vi "ProjectionExp_H.vi"() -> ()   [LabVIEW 2017]
uses:
  <vilib>/gmath/statdist.llb/Random Permutation.vi
  <instrlib>/Tektronix TDS 200 1000 2000 Series/Tektronix TDS 200 1000 2000 Series.lvlib
  <vilib>/gmath/NI_Gmath.lvlib
panel:
  out "RandRows":i32[](array[numeric])
  out "Bernoulli random numbers":u32[](array[numeric])
  out "error 2":i32
  in  "reset":bool
  in  "seed":i32=-1
  out "Phi zeros":dbl[][](array[numeric])
  out "x2 zeros":dbl[][](array[numeric])
  out "x1 zeros":dbl[][](array[numeric])
  in  "n":i32
  out "Theta zeros":dbl[][](array[numeric])
  in  "m":i32
  out "y zeros":dbl[][](array[numeric])
  out "error out 3":errorcluster caption="error out"
  in  "Delay Time (s) 2":dbl=1.0 caption="Delay Time (s)"
  in  "error in (no error) 3":errorcluster caption="error in (no error)"
  out "error out 2":errorcluster caption="error out"
  in  "Delay Time (s)":dbl=1.0
  in  "error in (no error) 2":errorcluster caption="error in (no error)"
  out "Iteration":i32
  out "Phi":dbl[][](array[numeric])
  out "y (Measurement \nMatrix)":dbl[][](array[numeric])
  out "VISA resource name out":refnum<visa-resource-name>
  out "Measurement":dbl
  out "Units":string
  out "error out":errorcluster
  in  "VISA resource name":refnum<visa-resource-name>
  in  "Channel (1: Channel 1)":i32(ring)=1 items=["Channel 1"=1, "Channel 2"=2, "Channel 3"=3, "Channel 4"=4]
  in  "Measurement Type (0: Frequency)":i32(ring) items=["Frequency", "Mean", "Period", "Pulse Duty", "Peak to Peak", "Cycle RMS", "Minimum", "Maximum", "Rise Time", "Fall Time", "Positive Width", "Negative Width", "Amplitude", "Cycle Mean", "High", "Low", "Negative Duty", "Positive Overshoot", "Negative Overshoot", "Cursor Mean", "Burst Width", "Positive Pulse Count", "Negative Pulse Count", "Rising Edge Count", "Falling Edge Count", "Area", "Cycle Area", "RMS", "Cursor RMS"]
  in  "error in (no error)":errorcluster
  out "Theta":dbl[][](array[numeric])
  in  "k":dbl
  in  "m":dbl
  in  "n":dbl
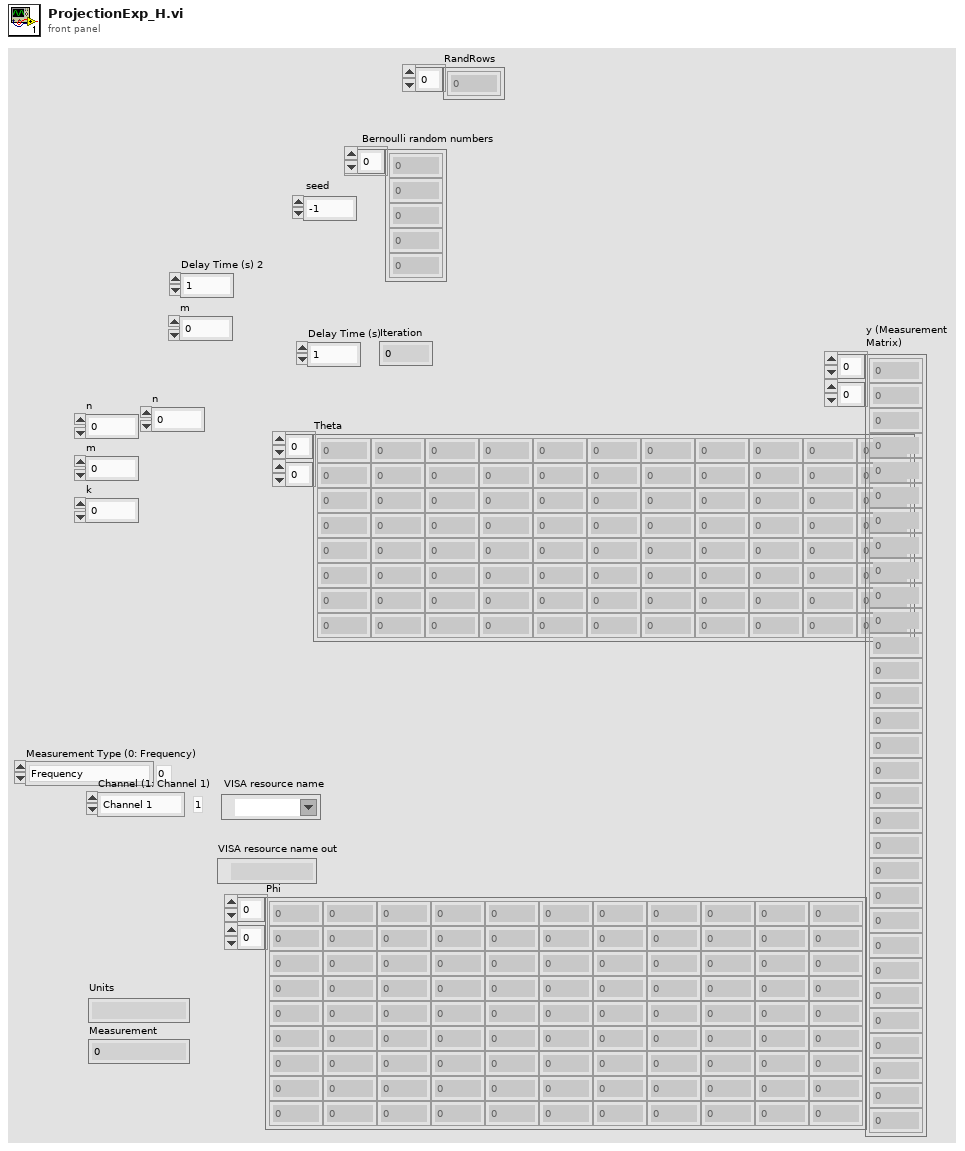
[diagram p1: front panel]
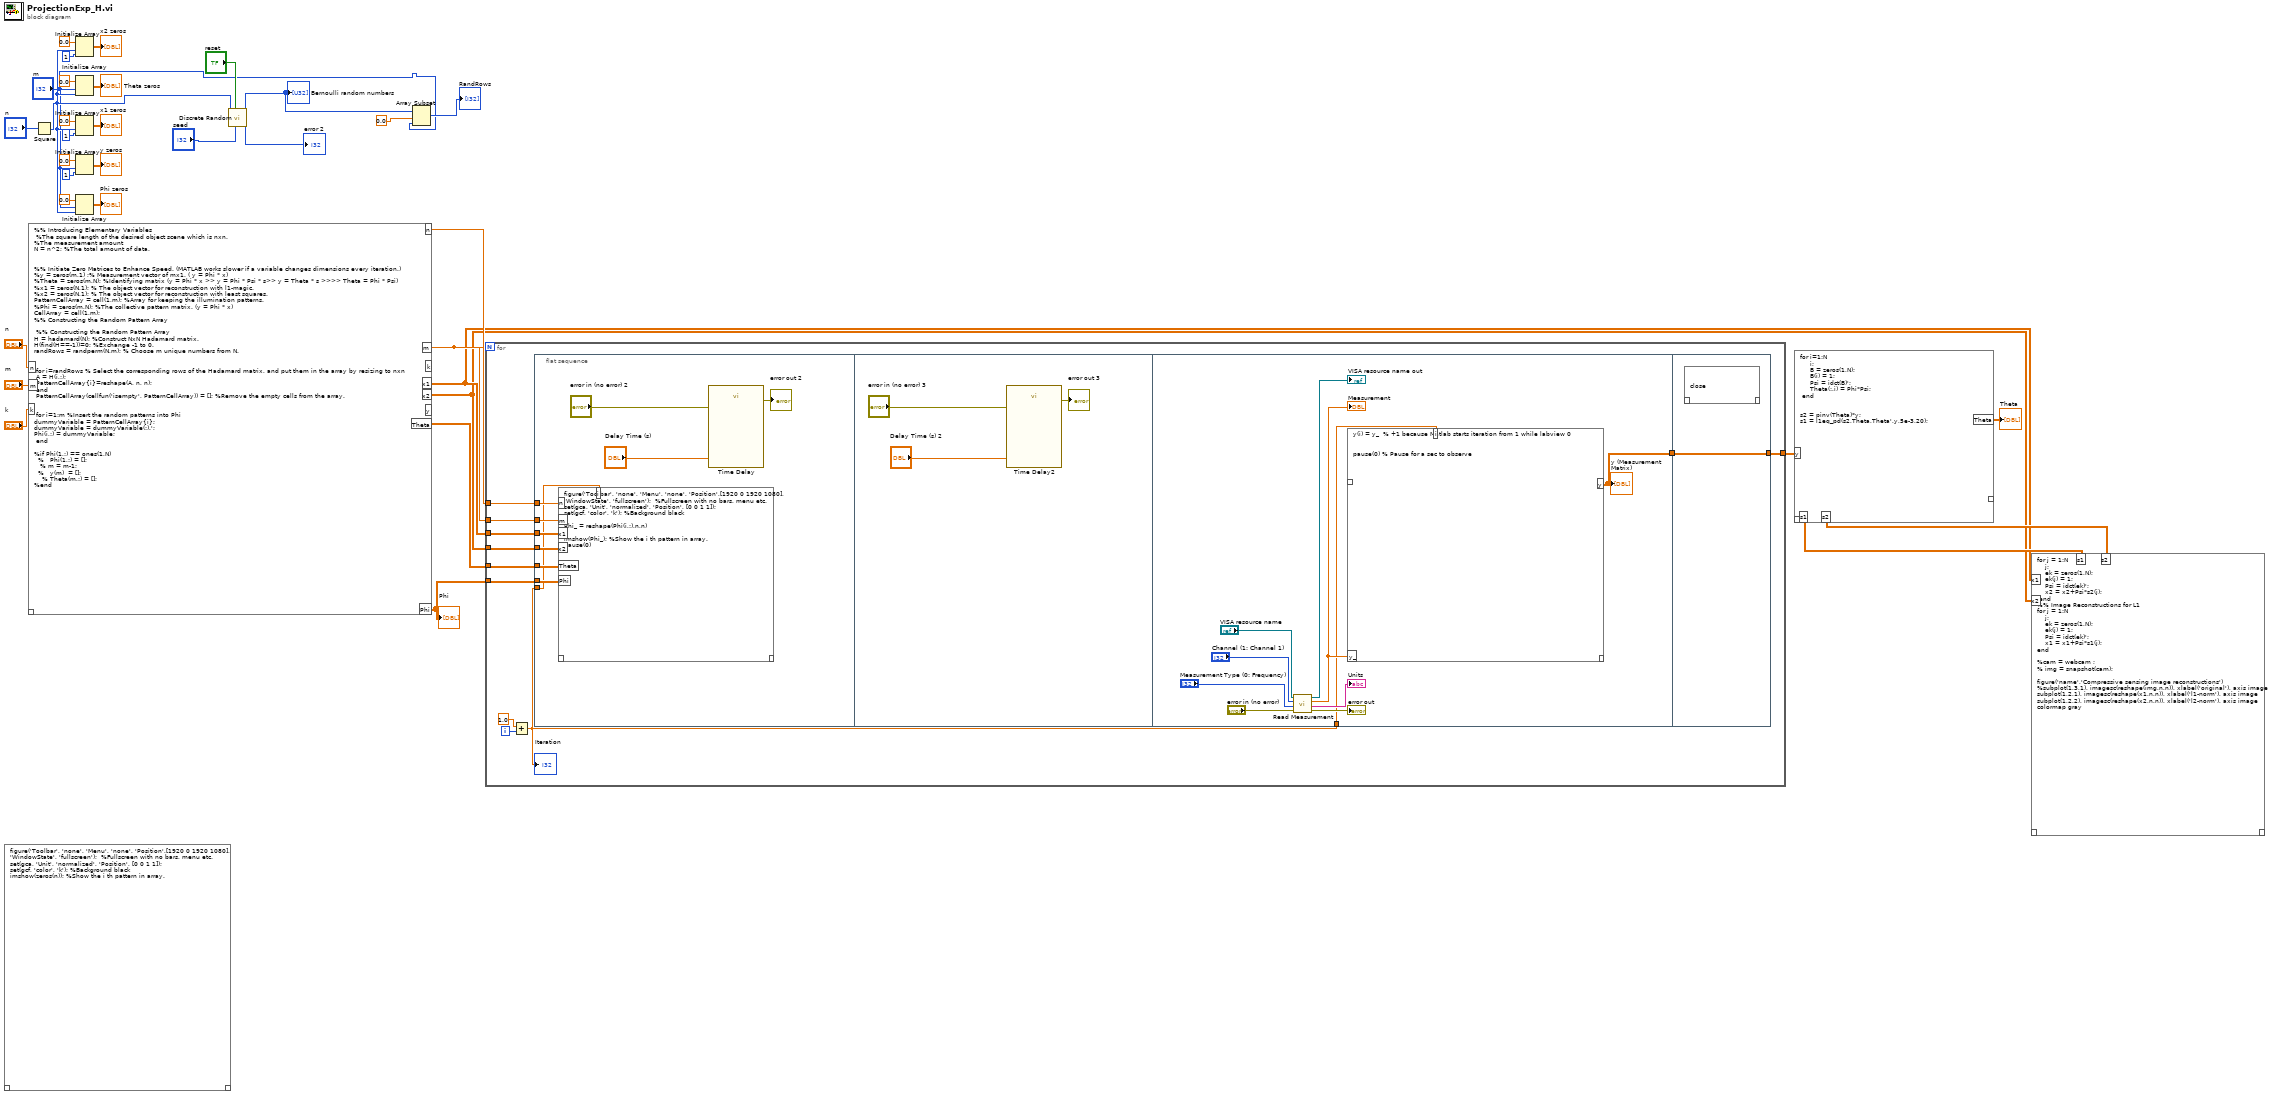
[diagram p0: block diagram]
diagram:
  n1 = script code="figure('Toolbar', 'none', 'Menu', 'none', 'Position',[1920 0 1920 1080], 'WindowState', 'fullscreen');  %Fullscreen with no bars, menu etc.\nset(gca, 'Unit', 'normalized', 'Position', [0 0 1 1]);\nset(gcf, 'color', 'k'); %Background black\nimshow(zeros(n)); %Show the i th pattern in array."() -> ()  [unwired: 1 in, 1 out]
  n2 = script code="%% Introducing Elementary Variables\n %The square length of the desired object scene which is nxn. \n%The measurement amount\nN = n^2; %The total amount of data. \n\n\n%% Initiate Zero Matrices to Enhance Speed. (MATLAB works slower if a variable changes dimensions every iteration.)\n%y = zeros(m,1) ;% Measurement vector of mx1. ( y = Phi * x)\n%Theta = zeros(m,N); %Identifying matrix (y = Phi * x >> y = Phi * Psi * s>> y = Theta * s >>>> Theta = Phi * Psi)\n%x1 = zeros(N,1); % The object vector for reconstruction with l1-magic.\n%x2 = zeros(N,1); % The object vector for reconstruction with least squares.\nPatternCellArray = cell(1,m); %Array for keeping the illumination patterns.\n%Phi = zeros(m,N); %The collective pattern matrix. (y = Phi * x)\nCellArray = cell(1,m);\n%% Constructing the Random Pattern Array\n\n %% Constructing the Random Pattern Array\nH = hadamard(N); %Construct NxN Hadamard matrix. \nH(find(H==-1))=0; %Exchange -1 to 0.\nrandRows = randperm(N,m); % Choose m unique numbers from N.\n\n\n for i=randRows % Select the corresponding rows of the Hadamard matrix, and put them in the array by resizing to nxn\n A = H(i,:);\n PatternCellArray{i}=reshape(A, n, n);\n end\n PatternCellArray(cellfun('isempty', PatternCellArray)) = []; %Remove the empty cells from the array.\n\n\n for i=1:m %Insert the random patterns into Phi\ndummyVariable = PatternCellArray{i}; \ndummyVariable = dummyVariable(:).';\nPhi(i,:) = dummyVariable;\n end\n\n%if Phi(1,:) == ones(1,N)\n  %   Phi(1,:) = [];\n   % m = m-1;\n  %   y(m)  = []; \n    % Theta(m,:) = [];\n%end"("n"="n", "m"="m", "k"="k") -> ("n"=w28:dbl, "m"=w27:dbl, "Phi"=w23:dbl[][], "Theta"=w24:dbl[][], "x1"=w26:dbl[][], "x2"=w25:dbl[][])  [unwired: 1 in, 3 out]
  "Phi" <- w23
  n3 = Square(x="n") -> (x^2=w5:i32)
  n4 = Initialize Array(0.0 ("element"), w5, 1 ("dimension size")) -> (→"x2 zeros":dbl[][])
  n5 = Initialize Array(0.0 ("element"), "m", w5) -> (→"Theta zeros":dbl[][])
  n6 = Initialize Array(0.0 ("element"), w5, 1 ("dimension size")) -> (→"x1 zeros":dbl[][])
  n7 = Initialize Array(0.0 ("element"), "m", 1 ("dimension size")) -> (→"y zeros":dbl[][])
  n8 = Initialize Array(0.0 ("element"), "m", w5) -> (→"Phi zeros":dbl[][])
  n9 = call-poly <vilib>:"Discrete Random.vi"("seed"="seed", "reset"="reset", "N"=w5) -> ("error"=→"error 2":i32, "random permutation"=w4:i32[])  [unwired: 7 in]
  "Bernoulli random numbers" <- w4
  n10 = Array Subset(array=w4, index=0.0 ("element"), length="m") -> (→"RandRows":i32[])
  n11 = for {
    N: w27 -> [_]
    tunnel: [w46] -> w29
    tunnel: w28 -> [w45]
    tunnel: w27 -> [w44]
    tunnel: w26 -> [w43]
    tunnel: w25 -> [w42]
    tunnel: w24 -> [w41]
    tunnel: w23 -> [w40]
    i -> [w37]
    n12 = Add(x=1.0, y=w37) -> (x+y=w36:dbl)
    "Iteration" <- w36
    n13 = flat-sequence {
      tunnel: w45 -> [w56]
      tunnel: w44 -> [w55]
      tunnel: w43 -> [w54]
      tunnel: w42 -> [w53]
      tunnel: w41 -> [w52]
      tunnel: w40 -> [w51]
      tunnel: w36 -> [w50]
      tunnel: w36 -> [w60]
      tunnel: [w61] -> w39
      tunnel: [w70] -> w46
      tunnel: w39 -> [w70]
      frame #0 {
        n14 = script code="figure('Toolbar', 'none', 'Menu', 'none', 'Position',[1920 0 1920 1080], 'WindowState', 'fullscreen');  %Fullscreen with no bars, menu etc.\nset(gca, 'Unit', 'normalized', 'Position', [0 0 1 1]);\nset(gcf, 'color', 'k'); %Background black\n\nPhi_ = reshape(Phi(i,:),n,n)\n\nimshow(Phi_); %Show the i th pattern in array. \npause(0)"("n"=w56, "m"=w55, "x1"=w54, "x2"=w53, "Theta"=w52, "Phi"=w51, "i"=w50) -> ()  [unwired: 1 in, 1 out]
        n15 = call "Time Delay"("error in (no error)"="error in (no error) 2", "Delay Time (s)"="Delay Time (s)") -> ("error out"=→"error out 2":errorcluster)  [unwired: 9 in]
      }
      frame #1 {
        n16 = call "Time Delay2"("error in (no error)"="error in (no error) 3", "Delay Time (s)"="Delay Time (s) 2") -> ("error out"=→"error out 3":errorcluster)  [unwired: 9 in]
      }
      frame #2 {
        n17 = call <instrlib>:"Read Measurement.vi"("error in (no error)"="error in (no error)", "Measurement Type (0: Frequency)"="Measurement Type (0: Frequency)", "Channel (1: Channel 1)"="Channel (1: Channel 1)", "VISA resource name"="VISA resource name") -> ("error out"=→"error out":errorcluster, "Units"=→"Units":string, "Measurement"=w69:dbl, "VISA resource name out"=→"VISA resource name out":refnum<visa-resource-name>)  [unwired: 4 in]
        "Measurement" <- w69
        n18 = script code="y(i) = y_  % +1 because Matlab starts iteration from 1 while labview 0 \n\n\npause(0) % Pause for a sec to observe"("i"=w60, "y_"=w69) -> ("y"=w61:dbl[][])  [unwired: 1 in, 1 out]
        "y (Measurement \nMatrix)" <- w61
      }
      frame #3 {
        n19 = script code="close"() -> ()  [unwired: 1 in, 1 out]
      }
    }
  }
  n20 = script code="for i=1:N\n     i;\n     B = zeros(1,N);\n     B(i) = 1;\n     Psi = idct(B)';\n     Theta(:,i) = Phi*Psi;    \n end\n\n\ns2 = pinv(Theta)*y;\ns1 = l1eq_pd(s2,Theta,Theta',y,5e-3,20);"("y"=w29) -> ("Theta"=→"Theta":dbl[][], "s1"=w31:dbl[][], "s2"=w30:dbl[][])  [unwired: 1 in, 1 out]
  n21 = script code="for j = 1:N\n    j;\n    ek = zeros(1,N);\n    ek(j) = 1;\n    Psi = idct(ek)';\n    x2 = x2+Psi*s2(j);\n end\n%% Image Reconstructions for L1\nfor j = 1:N\n    j;\n    ek = zeros(1,N);\n    ek(j) = 1;\n    Psi = idct(ek)';\n    x1 = x1+Psi*s1(j);\nend\n\n%cam = webcam ;\n% img = snapshot(cam);\n\nfigure('name','Compressive sensing image reconstructions')\n%subplot(1,3,1), imagesc(reshape(img,n,n)), xlabel('original'), axis image\nsubplot(1,2,1), imagesc(reshape(x1,n,n)), xlabel('l1-norm'), axis image\nsubplot(1,2,2), imagesc(reshape(x2,n,n)), xlabel('l2-norm'), axis image\ncolormap gray"("s1"=w31, "s2"=w30, "x2"=w25, "x1"=w26) -> ()  [unwired: 1 in, 1 out]
